vi "ExampleIVsweep.vi"() -> ()   [LabVIEW 2021]
panel:
  in  "Dwell time (ms)":u32
  in  "Vstop":dbl=1.0
  in  "Vstart":dbl
  in  "Npoints":i32=20
  out "IV Curve":cluster{"Voltage":dbl[], "Current":sgl[]}(graph)
  in  "Port":refnum<visa-resource-name>
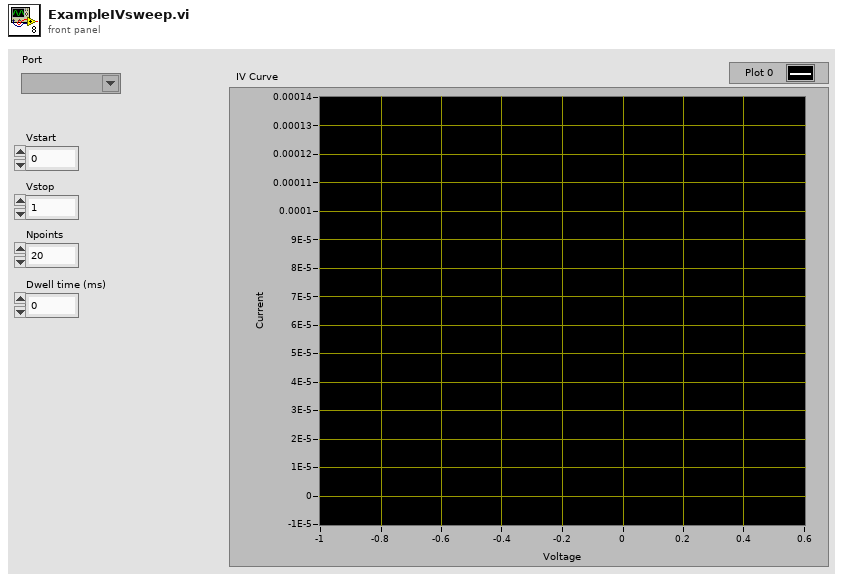
[diagram p1: front panel]
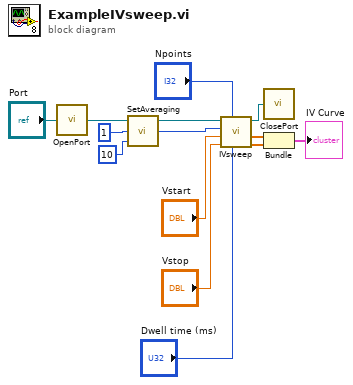
[diagram p0: block diagram]
diagram:
  n1 = call "OpenPort.vi"("Port"="Port") -> ("Serial port"=w13:refnum<visa-resource-name>)
  n2 = call "SetAveraging.vi"("Averages"=10, "Device"=u8 1, "Serial port"=w13) -> ("Device out"=w9:u8, "Serial port out"=w10:refnum<visa-resource-name>)  [unwired: 1 in]
  n3 = call "IVsweep.vi"("Dwell time"="Dwell time (ms)", "Npoints"="Npoints", "Vstop"="Vstop", "Vstart"="Vstart", "Device"=w9, "Serial port"=w10) -> ("Current"=w2:sgl[], "Voltage"=w3:dbl[], "Serial port out"=w8:refnum<visa-resource-name>)  [unwired: 1 out]
  n4 = call "ClosePort.vi"("Serial port"=w8) -> ()  [unwired: 1 in]
  n5 = Bundle("Voltage"=w3, "Current"=w2) -> (→"IV Curve":cluster{"Voltage":dbl[], "Current":sgl[]})  [unwired: 1 in]
